vi "PCP Interface Loop control and com settign.vi"(1 "Action(GET)":T1, 7 "Anytjhing":variant, 11 "error in (no error)":errorcluster) -> (6 "Run Command":bool, 8 "Comport out":refnum<visa-resource-name>, 10 "Running?":bool, 15 "error out":errorcluster)   [LabVIEW 2010]
uses:
  PCP return data types/PCP Interrface Loop control Action.ctl
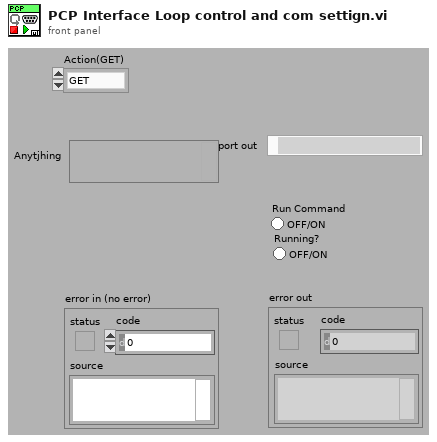
[diagram p1: front panel]
types:
  T1 = typedef "PCP Interrface Loop control Action.ctl" = enum16{"GET", "SET Comport", "SET Run!", "SET Runnig"}
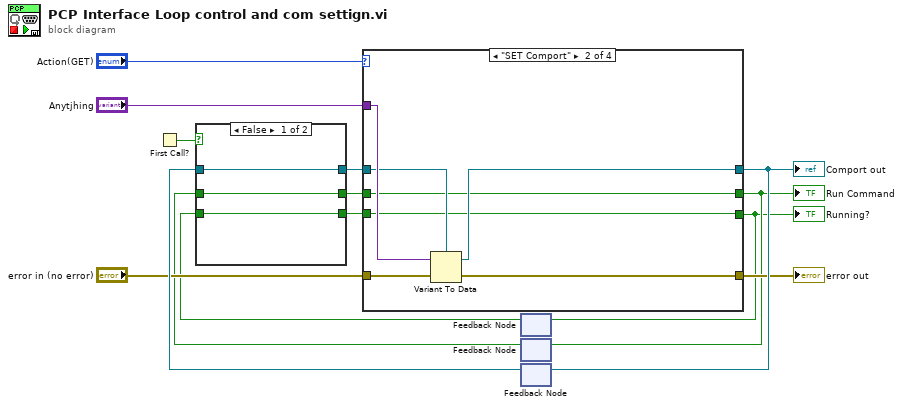
[diagram p0: block diagram]
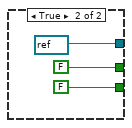
[diagram p2: hidden frame]
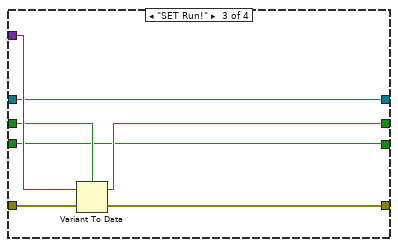
[diagram p4: hidden frame]
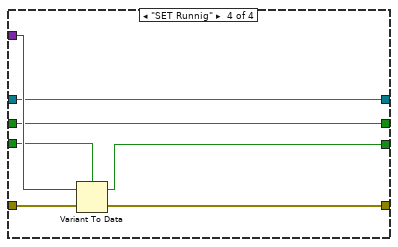
[diagram p5: hidden frame]
diagram:
  n1 = First Call?() -> (First Call?: T/F=w12:bool)
  n2 = feedback #1() -> (w1:bool)  [unwired: 1 in]
  n3 = feedback #2() -> (w4:bool)  [unwired: 1 in]
  n4 = feedback #3() -> (w13:refnum<visa-resource-name>)  [unwired: 1 in]
  n5 = case shown="False" w12 {
    tunnel: w13 -> [w17 _]
    tunnel: [w17 refnum<visa-resource-name> refnum ("Comport")] -> w10
    tunnel: [w15 FALSE] -> w6
    tunnel: w4 -> [w15 _]
    tunnel: [w16 FALSE] -> w3
    tunnel: w1 -> [w16 _]
    frame False {
    }
    frame True {
    }
  }
  n6 = case shown="\"SET Comport\"" "Action(GET)" {
    tunnel: [w24 w27 w35 w42] -> w11
    tunnel: w10 -> [w24 w28 w35 w42]
    tunnel: "Anytjhing" -> [_ w29 w36 w43]
    tunnel: [w23 w30 w37 w44] -> w8
    tunnel: "error in (no error)" -> [w23 w31 w38 w45]
    tunnel: w6 -> [w22 w26 w34 w41]
    tunnel: [w22 w26 w33 w41] -> w5
    tunnel: w3 -> [w21 w25 w32 w40]
    tunnel: [w21 w25 w32 w39] -> w2
    frame "GET", Default {
    }
    frame "SET Comport" {
      n7 = Variant To Data(error in=w31, Variant=w29, type=w28) -> (error out=w30:errorcluster, data=w27:refnum<visa-resource-name>)
    }
    frame "SET Run!" {
      n8 = Variant To Data(error in=w38, Variant=w36, type=w34) -> (error out=w37:errorcluster, data=w33:bool)
    }
    frame "SET Runnig" {
      n9 = Variant To Data(error in=w45, Variant=w43, type=w40) -> (error out=w44:errorcluster, data=w39:bool)
    }
  }
  "error out" <- w8
  "Comport out" <- w11
  "Run Command" <- w5
  "Running?" <- w2
  n10 = feedback-in #1(w2) -> ()
  n11 = feedback-in #2(w5) -> ()
  n12 = feedback-in #3(w11) -> ()
